vi "Read Serial.vi"(8 "error in (no error)":errorcluster, 11 "ThAr in":refnum<class "ThAr.lvclass">) -> (0 "error out":errorcluster, 2 "Serial":string, 3 "ThAr out":refnum<class "ThAr.lvclass">)   [LabVIEW 2016, in "ThAr.lvclass"]
uses:
  ThAr.lvclass
  ThAr.lvclass/ThAr.ctl
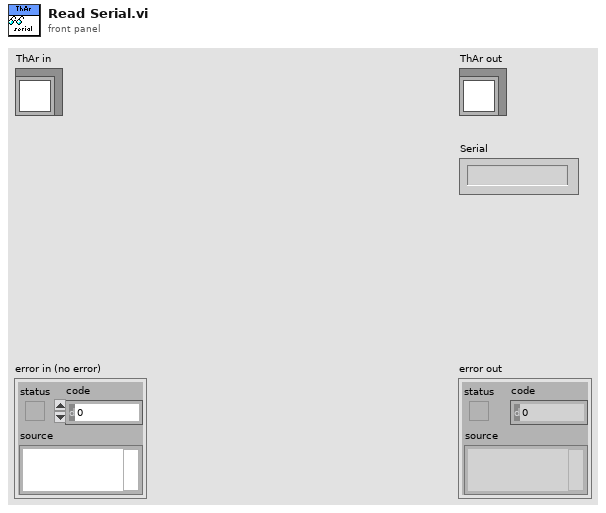
[diagram p1: front panel]
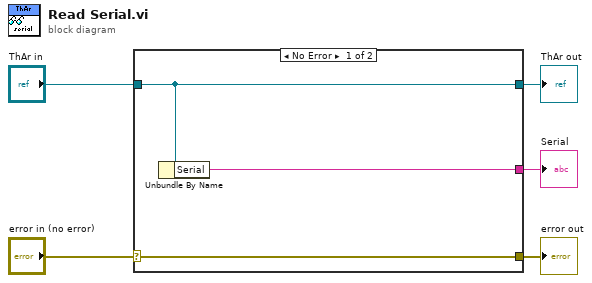
[diagram p0: block diagram]
diagram:
  n1 = case shown="No Error" "error in (no error)" {
    selector: "error in (no error)" -> [w8 w9]
    tunnel: [w8 w9] -> w4
    tunnel: [w7 w10] -> w2
    tunnel: "ThAr in" -> [w7 w10]
    tunnel: [w6 _] -> w1
    frame No Error {
      n2 = Unbundle By Name(w7) -> ("Serial"=w6:string)
    }
    frame Error {
    }
  }
  "error out" <- w4
  "ThAr out" <- w2
  "Serial" <- w1
